vi "ni579x FPGA Align.vi"(0 "sync.resources":T1, 1 "sync.meas.Reference Clock":refnum<k21>, 2 "sync.meas.FPGA Clock x2":refnum<k21>) -> (4 "sync.resources":T1)   [LabVIEW 2015, in "ni579x Synchronization v1 FPGA.lvlib"]
doc: "*** THIS VI IS DEPRECATED. USE ni579x FPGA Align 2.vi ***\n\nAlign the targets participating in synchronization. This must occur before a signal can be synchronized.\n\nThere are two flavors of alignment to chose from -- Host Align and FPGA Align. The two flavors produce the same quality of synchronization, but differ in requirements and versatility of operation.\n\nWhen using <B>ni579x FPGA Align</B>, the Single Cycle Timed Loop (SCTL) rate (that this VI is in) must be an integer multiple of the <B>sync.cptr.Reference Clock</B> rate, and the SCTL clock must have a fixed phase relationship to the reference clock. Each target performs its alignment independently, so FPGA Align does not require an FPGA I/O line. It's also possible to use FPGA Align without host interaction. FPGA Align has 100% repeatability if-and-only-if the target-to-target phase relationship is low and does not change.\n\nWhen using <B>ni579x Host Align</B>, the SCTL rate may be arbitrary (yet still must have a fixed phase relationship to the other targets). The CPTR period may also be arbitrary. This alignment process is coordinated by the host, and requires an FPGA I/O line for orchestration. Host Align has 100% repeatability; if the hardware configuration remains constant, so will the level of synchronization.\n\n<B>Input Parameters</B>\n\n<B>sync.resources</B> identifies the Synchronization instance. 'sync.resources' is obtained from the ni579x Create VI of this library.\n\n<B>sync.meas.Reference Clock</B> is used by the measurement logic as the \"start\" signal.\n\nWhen using 'ni579x FPGA Align', the 'sync.meas.Reference Clock' must be the same clock that the target's FPGA Clock is locked to. This is commonly PXI_Clk10.\n\n<B>sync.meas.FPGA Clock x2</B> is used by the measurement logic as the measurement clock. This clock must run at twice the rate of the FPGA Clock (the clock that drives the Single Cycle Timed Loop (SCTL) which this VI is in). This clock must also be derrived from the FPGA Clock, so that it has a fixed phase relationship. This is commonly IO Module\\Sample Clock x2.\n\n<B>Output Parameters</B>\n\n<B>sync.resources</B> is the same instance that was passed in for 'sync.resources'."
uses:
  <instrlib>/ni579x/Synchronization/v1/FPGA/ni579x Synchronization v1 FPGA.lvlib
  <vilib>/eio/EIONode/EIONode.xnode
  <instrlib>/_niInstr/TDC/v1/FPGA/niInstr Overclocked TDC v1 FPGA.lvlib
  <instrlib>/_niInstr/Basic Elements/v1/FPGA/niInstr Basic Elements v1 FPGA.lvlib
  <vilib>/rvi/eio/common/nirviEmuTemplateMethod_errors.vi
  <instrlib>/ni579x/Synchronization/v1/FPGA/Implementation/Resources.ctl
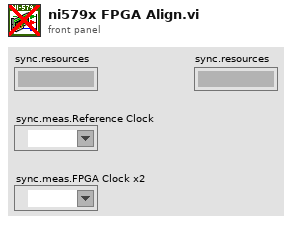
[diagram p1: front panel]
types:
  T1 = typedef "ni579x Synchronization v1 FPGA.lvlib/Resources.ctl" = cluster{"master":refnum<k21>, "meas.enable":refnum<k21>, "meas.ready":refnum<k21>, "meas.arm":refnum<k21>, "meas.valid":refnum<k21>, "meas.value":refnum<k21>, "meas.oversample clock":refnum<k21>, "meas.oversample factor":refnum<k21>, "cptr":refnum<k21>, "cptr.adjust":refnum<k21>, "cptr.period":refnum<k21>}
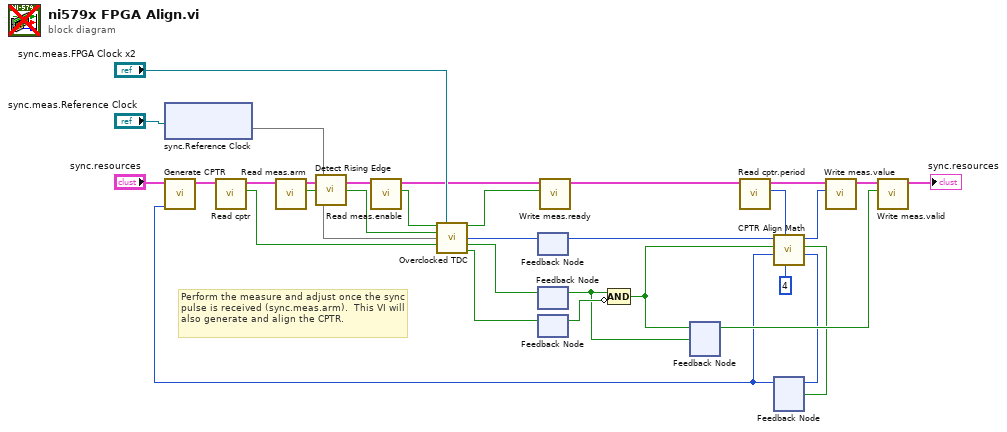
[diagram p0: block diagram]
diagram:
  # "Perform the measure and adjust once the sync pulse is received (sync.meas.arm).  This VI will also generate and align the CPTR."
  n1 = xnode ("sync.Reference Clock")("FPGA I/O In"="sync.meas.Reference Clock") -> ("I/O Item"=w8)  [unwired: 1 out]
  n2 = feedback #1() -> (w2:u16)  [unwired: 1 in]
  n3 = feedback #2() -> (w1:bool)  [unwired: 1 in]
  n4 = feedback #3() -> (w3:bool)  [unwired: 1 in]
  n5 = Compound Arithmetic op=AND(w1, invert w3) -> (w21:bool)
  n6 = feedback #4() -> (w31:bool)  [unwired: 1 in]
  n7 = feedback-in #4(w21, w1) -> ()
  n8 = feedback #5() -> (w25:u16)  [unwired: 1 in]
  n9 = call <instrlib>:"Generate CPTR.vi"("sync.cptr.adjust"=w25, "sync.resources"="sync.resources") -> ("sync.resources"=w26:T1)  [unwired: 9 in]
  n10 = call <instrlib>:"Read cptr.vi"("sync.resources"=w26) -> ("cptr"=w27:bool, "sync.resources"=w28:T1)  [unwired: 9 in]
  n11 = call <instrlib>:"Read meas.arm.vi"("sync.resources"=w28) -> ("meas.arm"=w29:bool, "sync.resources"=w13:T1)  [unwired: 9 in]
  n12 = call <instrlib>:"Detect Rising Edge.vi"("signal"=w29) -> ("edge detected"=w9:bool)  [unwired: 14 in]
  n13 = call <instrlib>:"Read meas.enable.vi"("sync.resources"=w13) -> ("meas.enable"=w10:bool, "sync.resources"=w12:T1)  [unwired: 9 in]
  n14 = call <instrlib>:"Overclocked TDC.vi"("enable"=w10, "counter clock"="sync.meas.FPGA Clock x2", "arm"=w9, "start"=w8, "stop"=w27) -> ("ready"=w7:bool, "count"=w6:u16, "count valid"=w4:bool, "rollover"=w5:bool)  [unwired: 6 in, 1 out]
  n15 = feedback-in #1(w6) -> ()
  n16 = feedback-in #2(w4) -> ()
  n17 = feedback-in #3(w5) -> ()
  n18 = call <instrlib>:"Write meas.ready.vi"("meas.ready"=w7, "sync.resources"=w12) -> ("sync.resources"=w11:T1)  [unwired: 9 in]
  n19 = call <instrlib>:"Read cptr.period.vi"("sync.resources"=w11) -> ("cptr.period"=w19:u16, "sync.resources"=w20:T1)  [unwired: 9 in]
  n20 = call <instrlib>:"CPTR Align Math.vi"("sync.meas.oversample factor"=u16 4, "sync.cptr.period"=w19, "sync.cptr.adjust"=w25, "measurement valid"=w21, "measurement"=w2) -> ("new sync.cptr.adjust"=w24:u16, "new sync.cptr.adjust valid"=w17:bool, "measurement (in sample clocks)"=w22:u16)  [unwired: 4 in]
  n21 = feedback-in #5(w24, w17) -> ()
  n22 = call <instrlib>:"Write meas.value.vi"("meas.value"=w22, "sync.resources"=w20) -> ("sync.resources"=w23:T1)  [unwired: 9 in]
  n23 = call <instrlib>:"Write meas.valid.vi"("meas.valid"=w31, "sync.resources"=w23) -> ("sync.resources"=→"sync.resources":T1)  [unwired: 9 in]
